vi "Switch_Test.vi"() -> ()   [LabVIEW 2018, in "Switch.lvlib"]
uses:
  Switch.lvlib
panel:
  in  "停止":bool
  out "通道2":bool
  out "通道1":bool
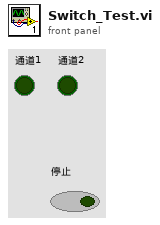
[diagram p1: front panel]
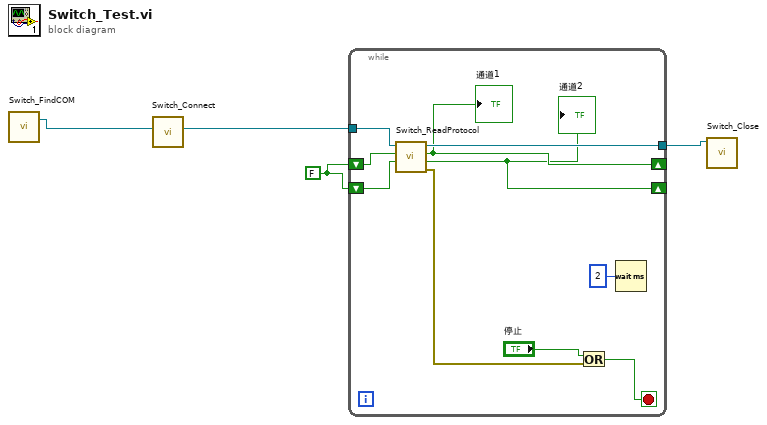
[diagram p0: block diagram]
diagram:
  w2 = FALSE
  n1 = call "Switch_FindCOM.vi"() -> ("VISA resource out"=w1:refnum<visa-resource-name>)  [unwired: 2 in, 1 out]
  n2 = call "Switch_Connect.vi"("COM"=w1) -> ("COM Out"=w4:refnum<visa-resource-name>)  [unwired: 9 in, 1 out]
  n3 = while {
    tunnel: w4 -> [w14]
    tunnel: [w13] -> w3
    shift-right: [w11] -> _
    shift-left: w2 -> [w9]
    shift-right: [w10] -> _
    shift-left: w2 -> [w8]
    stop <- w5 stop-if-true
    n4 = call "Switch_ReadProtocol.vi"("Old通道2"=w8, "Old通道1"=w9, "COM"=w14) -> ("错误输出"=w6:errorcluster, "通道2"=w10:bool, "通道1"=w11:bool, "COM Out"=w13:refnum<visa-resource-name>)  [unwired: 5 in]
    "通道2" <- w10
    "通道1" <- w11
    n5 = Or(x="停止", y=w6) -> (x .or. y?=w5:bool)
    n6 = Wait (ms)(milliseconds to wait=u32 2 ("等待时间（毫秒）")) -> ()  [unwired: 1 out]
  }
  n7 = call "Switch_Close.vi"("COM"=w3) -> ()  [unwired: 10 in, 1 out]
